vi "GetHostname.vi"(7 "LabVIEW Web Service Request":refnum<class "Web Request.lvclass">) -> ()   [LabVIEW 2015]
uses:
  <vilib>/wsapi/Web Request.lvclass
  <vilib>/addons/SystemInfoProcess/SystemInfoProcess.lvlib
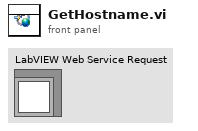
[diagram p1: front panel]
types:
  T1 = typedef "PointValueMap.lvlib/PointMap.ctl" = refnum<data-value>
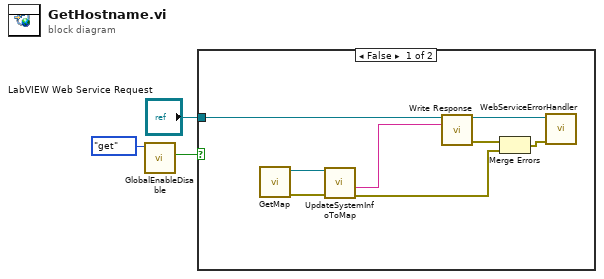
[diagram p0: block diagram]
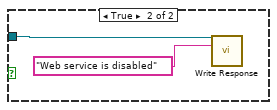
[diagram p2: hidden frame]
diagram:
  n1 = call "GlobalEnableDisable.vi"("action"=enum16{"init", "set", "get"}."get") -> ("DisableDeviceWebService"=w1:bool)  [unwired: 10 in]
  n2 = case shown="False" w1 {
    tunnel: "LabVIEW Web Service Request" -> [w11 w12]
    frame False {
      n3 = call <vilib>:"GetMap.vi"() -> ("error out"=w6:errorcluster, "SystemInfoMap"=w8:T1)  [unwired: 10 in]
      n4 = call <vilib>:"UpdateSystemInfoToMap.vi"("error in (no error)"=w6, "map in"=w8) -> ("error out"=w4:errorcluster, "hostname"=w7:string)  [unwired: 5 in, 3 out]
      n5 = call <vilib>:"Write Response.vi"("LabVIEW Web Service Request"=w11, "response string"=w7) -> ("LabVIEW Web Service Request out"=w10:refnum<class "Web Request.lvclass">, "error out"=w9:errorcluster)  [unwired: 12 in]
      n6 = Merge Errors(w9, w4) -> (w5:errorcluster)
      n7 = call "WebServiceErrorHandler.vi"("LabVIEW Web Service Request"=w10, "error in (no error)"=w5) -> ()  [unwired: 12 in, 2 out]
    }
    frame True {
      n8 = call <vilib>:"Write Response.vi"("LabVIEW Web Service Request"=w12, "response string"="Web service is disabled") -> ()  [unwired: 12 in, 2 out]
    }
  }
